vi "Example Graph.vi"() -> ()   [LabVIEW 2013]
uses:
  C:/tf/play/labview/Tinkerforge.dll
  Tinkerforge.dll
panel:
  in  "stop":bool
  out "graph":i32[](graph)
  in  "uid":string="amb"
  in  "port":i32=4223
  in  "host":string="localhost"
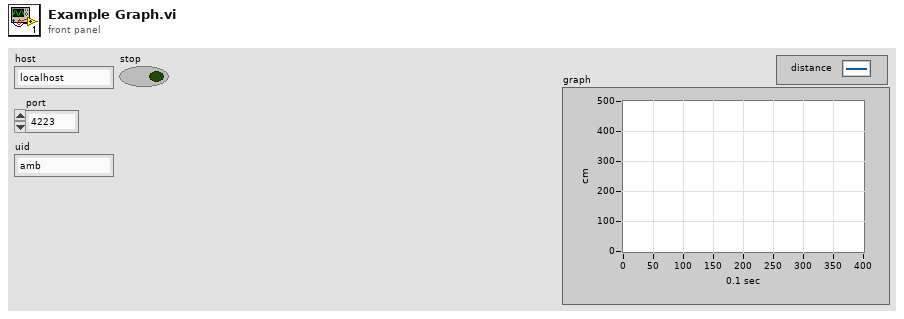
[diagram p1: front panel]
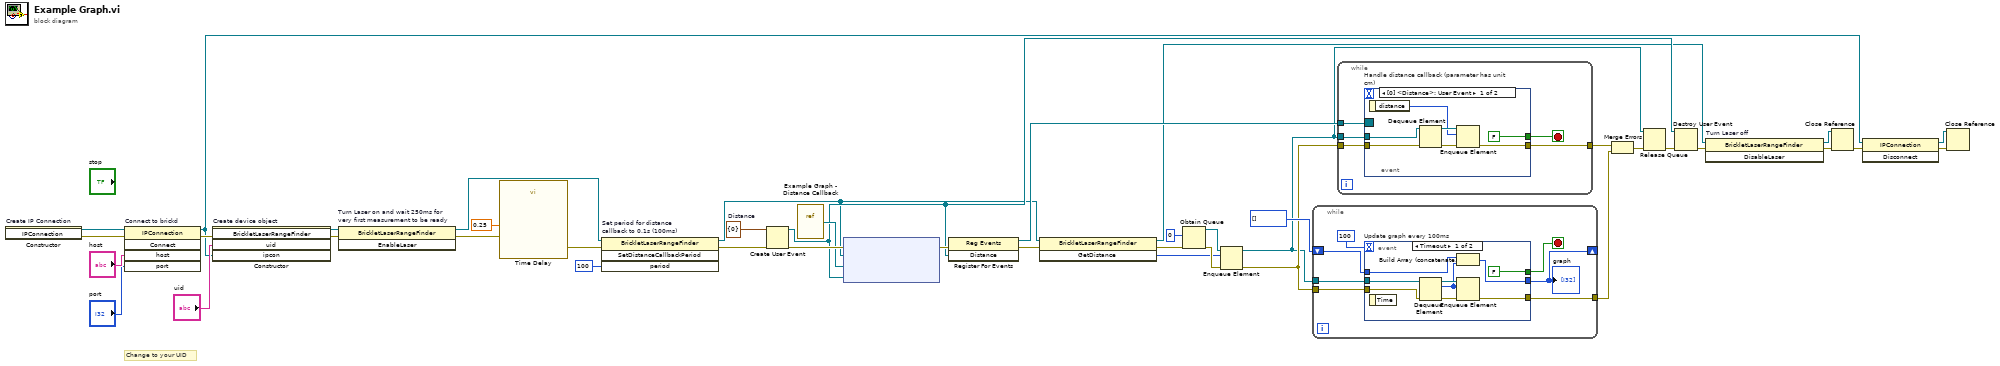
[diagram p0: block diagram]
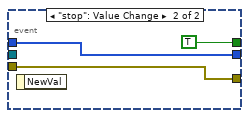
[diagram p2: hidden frame]
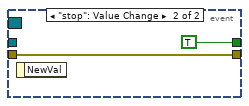
[diagram p3: hidden frame]
diagram:
  w28 = cluster{"distance":i32} {"distance"=0}  # Distance
  # "Change to your UID"
  n1 = constructor on="Create IP Connection" class="IPConnection"() -> (reference out=w42:refnum<k24>, error out=w15:errorcluster)  [unwired: 3 in, 1 out]
  n2 = invoke on="Connect to brickd" class="IPConnection" method="Connect"(reference=w42, error in=w15, "host"="host", "port"="port") -> (reference out=w35:refnum<k24>, error out=w38:errorcluster)  [unwired: 1 in, 3 out]
  n3 = constructor on="Create device object" class="BrickletLaserRangeFinder"(error in=w38, "uid"="uid", "ipcon"=w35) -> (reference out=w9:refnum<k24>, error out=w10:errorcluster)  [unwired: 2 in, 3 out]
  n4 = invoke on="Turn Laser on and wait 250ms for\nvery first measurement to be ready" class="BrickletLaserRangeFinder" method="EnableLaser"(reference=w9, error in=w10) -> (reference out=w8:refnum<k24>, error out=w6:errorcluster)  [unwired: 1 in, 1 out]
  n5 = call "Time Delay"("error in (no error)"=w6, "Delay Time (s)"=0.25) -> ("error out"=w5:errorcluster)  [unwired: 9 in]
  n6 = invoke on="Set period for distance\ncallback to 0.1s (100ms)" class="BrickletLaserRangeFinder" method="SetDistanceCallbackPeriod"(reference=w8, error in=w5, "period"=i64 100) -> (reference out=w12:refnum<k24>, error out=w27:errorcluster)  [unwired: 1 in, 2 out]
  n7 = Create User Event(user event datatype=w28, error in=w27) -> (user event=w29:refnum<user-event>, error out=w33:errorcluster)
  n8 = vi-ref "Example Graph - Distance Callback.vi"() -> ("vi reference"=w31:refnum<vi>)
  n9 = node ("Register Event Callback")(w33, w12, w31, w29) -> (w32:errorcluster)  [unwired: 1 in, 1 out]
  n10 = register-events(error in=w32, w29) -> (reference out=w30:refnum<event-registration>, error out=w14:errorcluster)  [unwired: 1 in]
  n11 = invoke class="BrickletLaserRangeFinder" method="GetDistance"(reference=w12, error in=w14) -> (reference out=w4:refnum<k24>, error out=w13:errorcluster, "GetDistance"=w11:i32)  [unwired: 1 in]
  n12 = Obtain Queue(element data type=0, error in (no error)=w13) -> (queue out=w19:refnum<queue>, error out=w21:errorcluster)  [unwired: 3 in, 1 out]
  n13 = Enqueue Element(queue=w19, element=w11, error in (no error)=w21) -> (queue out=w16:refnum<queue>, error out=w20:errorcluster)  [unwired: 1 in, 1 out]
  n14 = while {
    tunnel: [w45] -> w25
    tunnel: w20 -> [w46]
    shift-right: [w47] -> _
    shift-left: i32[] [] -> [w48]
    tunnel: w16 -> [w44]
    stop <- w43 stop-if-true
    n15 = event "Update graph every 100ms" shown="[0] Timeout" {
      selector: _ -> [_ _]
      dyn-events: _ -> [_ _]
      timeout: 100 -> [_ _]
      tunnel: [w58 w60] -> w47
      tunnel: w48 -> [w51 w60]
      tunnel: w46 -> [w57 w59]
      tunnel: [w54 w59] -> w45
      tunnel: w44 -> [w56 _]
      tunnel: [FALSE TRUE] -> w43
      event Timeout {
        n16 = event-data() -> ()  [unwired: 1 in, 1 out]
        n17 = Dequeue Element(queue=w56, error in (no error)=w57) -> (queue out=w53:refnum<queue>, element=w52:i32, error out=w55:errorcluster)  [unwired: 1 in, 1 out]
        n18 = Build Array (concatenate)(w51, w52) -> (w58:i32[])
        n19 = Enqueue Element(queue=w53, element=w52, error in (no error)=w55) -> (error out=w54:errorcluster)  [unwired: 1 in, 2 out]
      }
      event "stop": Value Change {
        n20 = event-data() -> ()  [unwired: 1 in, 1 out]
      }
    }
    "graph" <- w47
  }
  n21 = while {
    tunnel: w30 -> [w66]
    tunnel: [w64] -> w24
    tunnel: w20 -> [w65]
    tunnel: w16 -> [w63]
    stop <- w62 stop-if-true
    n22 = event "Handle distance callback (parameter has unit cm)" shown="[0] <Distance>: User Event" {
      selector: w66 -> [_ _]
      dyn-events: _ -> [_ _]
      timeout: _ -> [_ _]
      tunnel: w65 -> [w73 w74]
      tunnel: [w71 w74] -> w64
      tunnel: w63 -> [w70 _]
      tunnel: [FALSE TRUE] -> w62
      event User Event {
        n23 = event-data() -> ("distance"=w67:i32)  [unwired: 1 in]
        n24 = Dequeue Element(queue=w70, error in (no error)=w73) -> (queue out=w69:refnum<queue>, error out=w72:errorcluster)  [unwired: 1 in, 2 out]
        n25 = Enqueue Element(queue=w69, element=w67, error in (no error)=w72) -> (error out=w71:errorcluster)  [unwired: 1 in, 2 out]
      }
      event "stop": Value Change {
        n26 = event-data() -> ()  [unwired: 1 in, 1 out]
      }
    }
  }
  n27 = Merge Errors(w24, w25) -> (w18:errorcluster)
  n28 = Release Queue(queue=w16, error in (no error)=w18) -> (error out=w17:errorcluster)  [unwired: 1 in, 2 out]
  n29 = Destroy User Event(user event=w29, error in=w17) -> (error out=w2:errorcluster)
  n30 = invoke on="Turn Laser off" class="BrickletLaserRangeFinder" method="DisableLaser"(reference=w4, error in=w2) -> (reference out=w3:refnum<k24>, error out=w1:errorcluster)  [unwired: 1 in, 1 out]
  n31 = Close Reference(reference=w3, error in (no error)=w1) -> (error out=w37:errorcluster)
  n32 = invoke class="IPConnection" method="Disconnect"(reference=w35, error in=w37) -> (reference out=w34:refnum<k24>, error out=w36:errorcluster)  [unwired: 1 in, 1 out]
  n33 = Close Reference(reference=w34, error in (no error)=w36) -> ()  [unwired: 1 out]
